vi "Package Data.vi"(8 "error in":errorcluster, 10 "DataIn":string, 11 "Alicat Data in":refnum<class "Alicat Data.lvclass">) -> (0 "error out":errorcluster, 3 "Alicat Data out":refnum<class "Alicat Data.lvclass">)   [LabVIEW 2015, in "Alicat Data.lvclass"]
uses:
  Alicat Data.lvclass
  Reusable/Data/Write measTime.vi
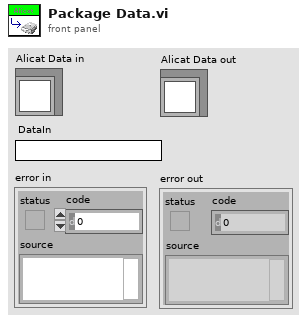
[diagram p1: front panel]
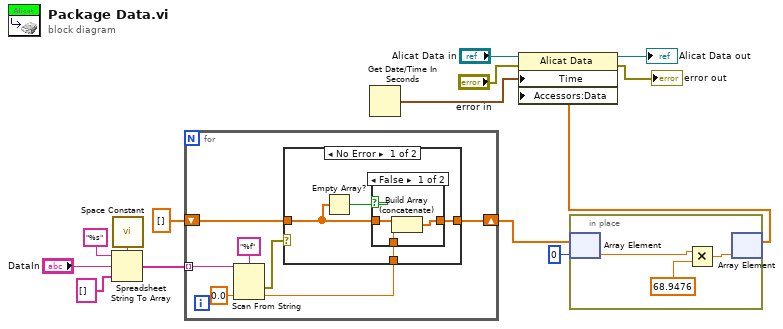
[diagram p0: block diagram]
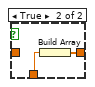
[diagram p2: hidden frame]
diagram:
  n1 = call <vilib>:"Space Constant.vi"() -> ("String"=w8:string)
  n2 = Spreadsheet String To Array(delimiter (Tab)=w8, format string="%s", spreadsheet string="DataIn", array type (2D Dbl)=string[] []) -> (array=w5:string[])
  n3 = for {
    tunnel: w5 -> [w21] mode=indexing
    shift-right: [w15] -> w3
    shift-left: sgl[] [] -> [w17]
    n4 = Scan From String(format string="%f", input string=w21, default 1=sgl 0.0) -> (error out=w18:errorcluster, output 1=w16:sgl)  [unwired: 2 in, 2 out]
    n5 = case shown="No Error" w18 {
      tunnel: w17 -> [w24 w31]
      tunnel: w16 -> [w23 _]
      tunnel: [w22 w31] -> w15
      frame No Error {
        n6 = Empty Array?(array=w24) -> (empty?=w25:bool)
        n7 = case shown="False" w25 {
          tunnel: w24 -> [w28 _]
          tunnel: w23 -> [w27 w30]
          tunnel: [w26 w29] -> w22
          frame False {
            n8 = Build Array (concatenate)(w28, w27) -> (w26:sgl[])
          }
          frame True {
            n9 = Build Array(w30) -> (w29:sgl[])
          }
        }
      }
      frame Error {
      }
    }
  }
  n10 = Get Date/Time In Seconds() -> (seconds since 1Jan1904=w12:timestamp)
  n11 = in-place {
    n12 = in-place-array #1(w3, 0) -> (w33:sgl)
    n13 = Multiply(x=w33, y=68.9476) -> (x*y=w32:dbl)
    n14 = in-place-array #1(w32) -> (w1:sgl[])  [unwired: 1 out]
  }
  n15 = property class="Alicat Data"(reference="Alicat Data in", error in="error in", "Time"=w12, "Accessors:Data"=w1) -> (reference out=→"Alicat Data out":refnum<class "Alicat Data.lvclass">, error out=→"error out":errorcluster)
